vi "Drive Call.vi"(1 "Joystick Axes":dbl[](array[numeric]), 2 "Right Button Values":bool[](array[boolean]), 3 "Left Button Values":bool[](array[boolean])) -> ()   [LabVIEW 2018]
uses:
  Implementation/Drive Setpoints.ctl
  Implementation/Drive Operations.ctl
  <vilib>/Rock Robotics/Network Tables/NT Write Boolean.vi
  <vilib>/functionblocks/Edge Detection/One Shot Rising with Input/One Shot Rising with Input.vi
  <vilib>/functionblocks/FB Core/FB Core.xnode
  <vilib>/functionblocks/NI_FunctionBlock Libraries.lvlib
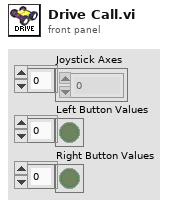
[diagram p1: front panel]
types:
  T1 = typedef "Drive Setpoints.ctl" = cluster{"Operation":T2, "Left Setpoint":dbl, "Right Setpoint":dbl, "Duration":dbl, "Enable Gyro Compensation":bool, "Gyro Turn Angle ":dbl}
  T2 = typedef "Drive Operations.ctl" = enum16{"Reserve", "Read Current", "Immediate", "Drive for Time", "Drive for Distance", "Gyro Turn"}
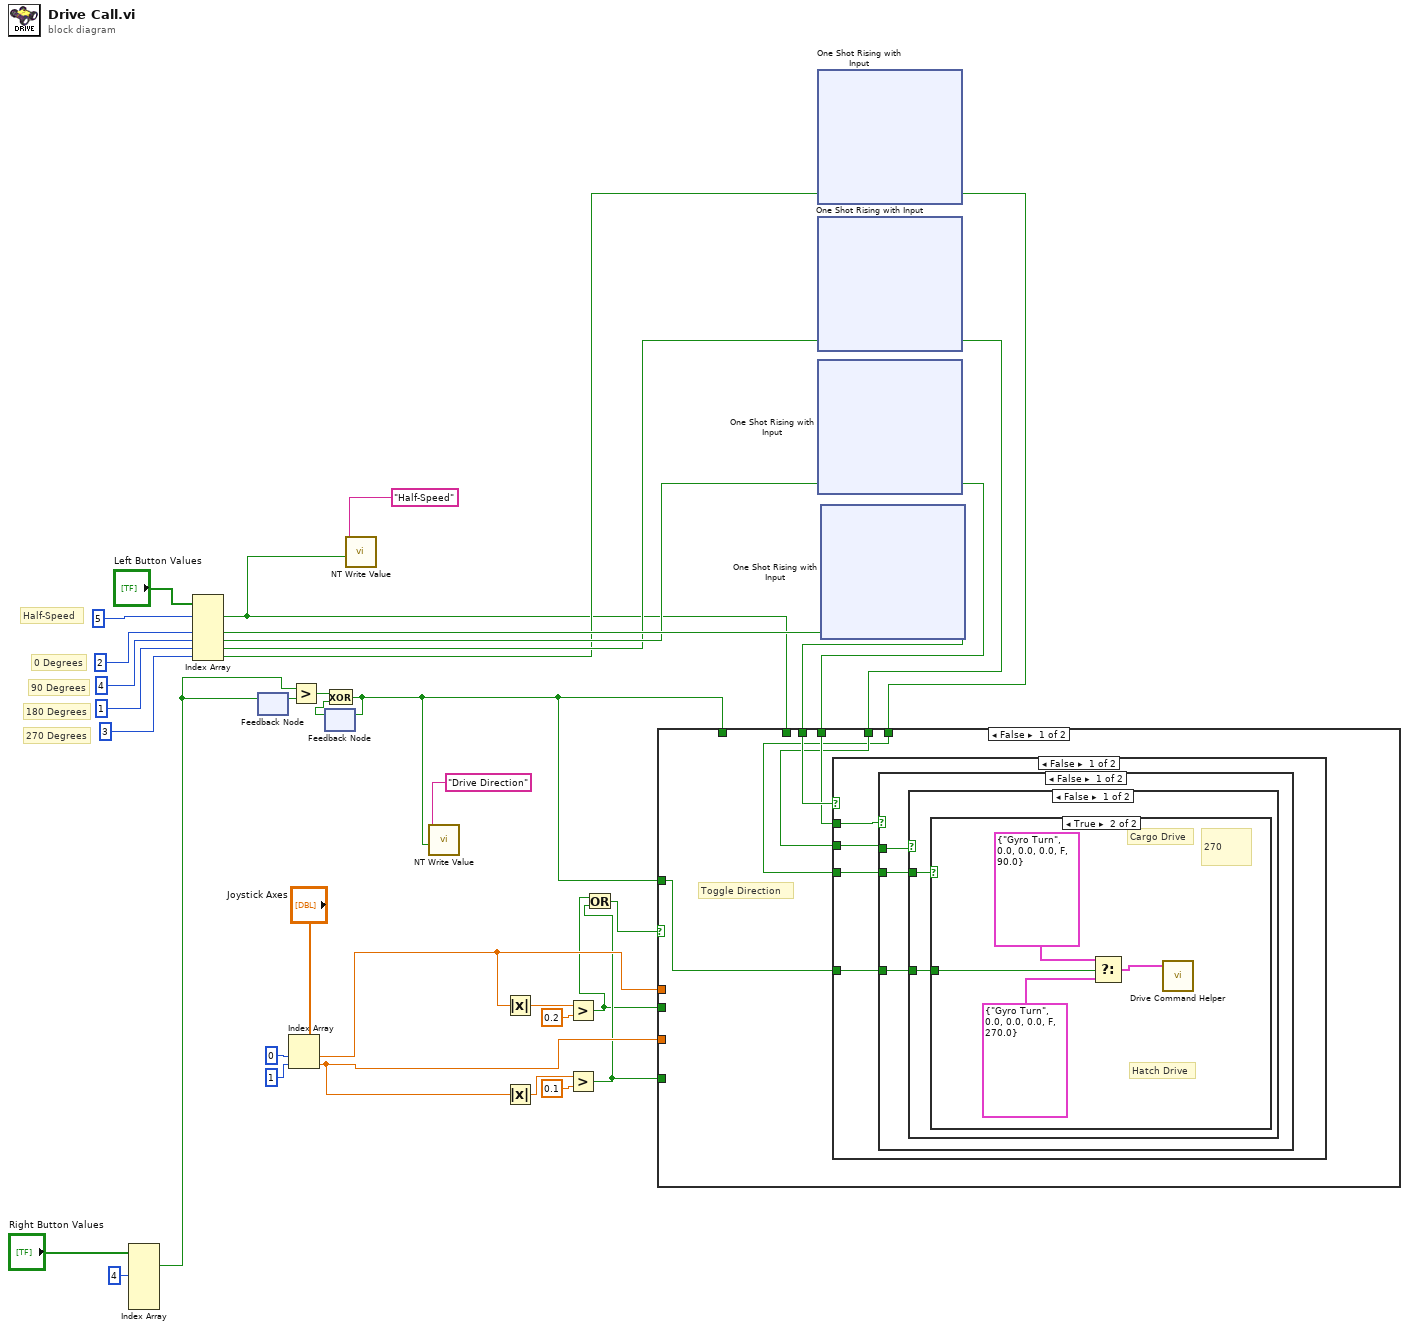
[diagram p0: block diagram]
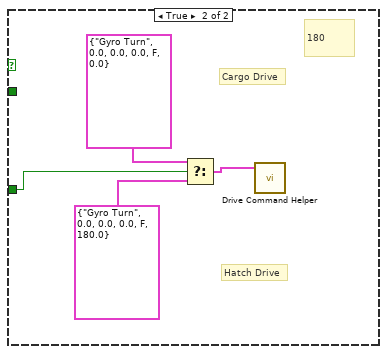
[diagram p3: hidden frame]
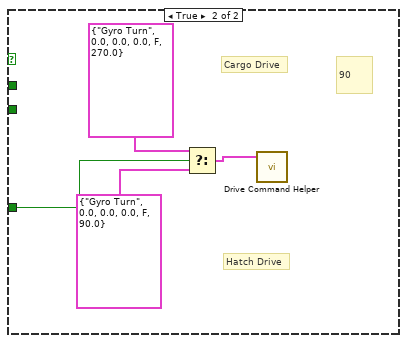
[diagram p4: hidden frame]
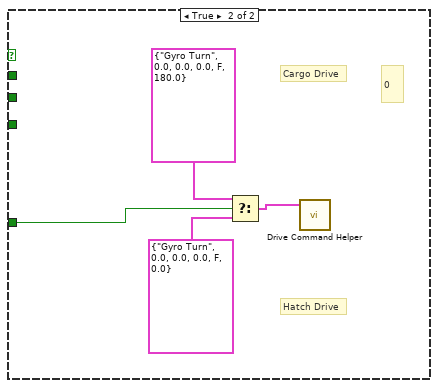
[diagram p5: hidden frame]
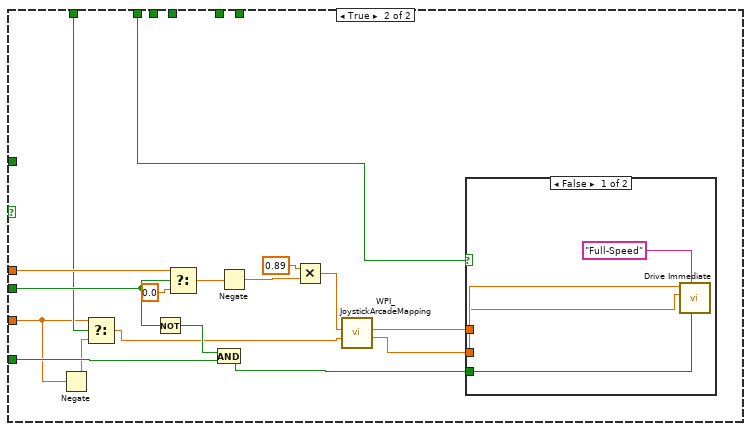
[diagram p6: hidden frame]
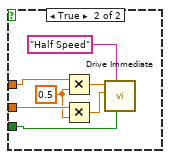
[diagram p7: hidden frame]
diagram:
  # "270 Degrees"
  # "180 Degrees"
  # "90 Degrees"
  # "0 Degrees"
  # "Half-Speed"
  n1 = Index Array(array="Right Button Values", index #1=4 ("index")) -> (element #1=w2:bool)  [unwired: 5 in, 5 out]
  n2 = Index Array(array="Left Button Values", index #1=5 ("index"), index #3=2 ("index"), index #4=4 ("index"), index #5=1 ("index"), index #6=3 ("index")) -> (element #1=w4:bool, element #3=w16:bool, element #4=w12:bool, element #5=w11:bool, element #6=w10:bool)  [unwired: 1 in, 1 out]
  n3 = feedback #1() -> (w25:bool)  [unwired: 1 in]
  n4 = feedback-in #1(w2) -> ()
  n5 = Index Array(array="Joystick Axes", index #1=0 ("index"), index #2=1 ("index")) -> (element #1=w27:dbl, element #2=w22:dbl)
  n6 = Greater?(x=w2, y=w25) -> (0:w26:bool)
  n7 = feedback #2() -> (w24:bool)  [unwired: 1 in]
  n8 = Exclusive Or(1:w24, 2:w26) -> (0:w9:bool)
  n9 = feedback-in #2(w9) -> ()
  n10 = call-poly <vilib>:"NT Write Value.vi"("Boolean"=w4, "Name"="Half-Speed") -> ()  [unwired: 9 in, 1 out]
  n11 = call-poly <vilib>:"NT Write Value.vi"("Boolean"=w9, "Name"="Drive Direction") -> ()  [unwired: 9 in, 1 out]
  n12 = Absolute Value(x=w27) -> (abs(x)=w31:dbl)
  n13 = Absolute Value(x=w22) -> (abs(x)=w29:dbl)
  n14 = Greater?(x=w31, y=0.2) -> (0:w20:bool)
  n15 = Greater?(x=w29, y=0.1) -> (0:w21:bool)
  n16 = Or(x=w20, y=w21) -> (x .or. y?=w19:bool)
  n17 = xnode "One Shot Rising with Input"("input"=w10) -> ("output"=w6:bool)  [unwired: 1 in, 1 out]
  n18 = xnode "One Shot Rising with Input"("input"=w11) -> ("output"=w7:bool)  [unwired: 1 in, 1 out]
  n19 = xnode "One Shot Rising with Input"("input"=w12) -> ("output"=w8:bool)  [unwired: 1 in, 1 out]
  n20 = xnode "One Shot Rising with Input"("input"=w16) -> ("output"=w17:bool)  [unwired: 1 in, 1 out]
  n21 = case shown="False" w19 {
    tunnel: w20 -> [_ w76]
    tunnel: w21 -> [_ w74]
    tunnel: w4 -> [_ w72]
    tunnel: w27 -> [_ w71]
    tunnel: w9 -> [_ w68]
    tunnel: w22 -> [_ w67]
    tunnel: w17 -> [w41 _]
    tunnel: w9 -> [w40 _]
    tunnel: w8 -> [w39 _]
    tunnel: w7 -> [w38 _]
    tunnel: w6 -> [w37 _]
    frame False {
      # "Toggle Direction"
      n22 = case shown="False" w41 {
        tunnel: w40 -> [w44 w63]
        tunnel: w39 -> [w45 _]
        tunnel: w38 -> [w43 _]
        tunnel: w37 -> [w42 _]
        frame False {
          n23 = case shown="False" w45 {
            tunnel: w44 -> [w48 w59]
            tunnel: w43 -> [w47 _]
            tunnel: w42 -> [w46 _]
            frame False {
              n24 = case shown="False" w47 {
                tunnel: w48 -> [w50 w55]
                tunnel: w46 -> [w49 _]
                frame False {
                  n25 = case shown="True" w49 {
                    tunnel: w50 -> [_ w51]
                    frame False {
                    }
                    frame True {
                      # "270"
                      # "Hatch Drive"
                      # "Cargo Drive"
                      n26 = Select(t=T1 {"Operation"=enum."Gyro Turn", "Left Setpoint"=0.0, "Right Setpoint"=0.0, "Duration"=0.0, "Enable Gyro Compensation"=FALSE, "Gyro Turn Angle "=90.0} ("SubSystem Data"), s=w51, f=T1 {"Operation"=enum."Gyro Turn", "Left Setpoint"=0.0, "Right Setpoint"=0.0, "Duration"=0.0, "Enable Gyro Compensation"=FALSE, "Gyro Turn Angle "=270.0} ("SubSystem Data")) -> (s? t:f=w53:T1)
                      n27 = call "Drive Command Helper.vi"("SubSystem Data"=w53) -> ()  [unwired: 8 in, 3 out]
                    }
                  }
                }
                frame True {
                  # "Hatch Drive"
                  # "Cargo Drive"
                  # "180"
                  n28 = Select(t=T1 {"Operation"=enum."Gyro Turn", "Left Setpoint"=0.0, "Right Setpoint"=0.0, "Duration"=0.0, "Enable Gyro Compensation"=FALSE, "Gyro Turn Angle "=0.0} ("SubSystem Data"), s=w55, f=T1 {"Operation"=enum."Gyro Turn", "Left Setpoint"=0.0, "Right Setpoint"=0.0, "Duration"=0.0, "Enable Gyro Compensation"=FALSE, "Gyro Turn Angle "=180.0} ("SubSystem Data")) -> (s? t:f=w57:T1)
                  n29 = call "Drive Command Helper.vi"("SubSystem Data"=w57) -> ()  [unwired: 8 in, 3 out]
                }
              }
            }
            frame True {
              # "Hatch Drive"
              # "Cargo Drive"
              # "90"
              n30 = Select(t=T1 {"Operation"=enum."Gyro Turn", "Left Setpoint"=0.0, "Right Setpoint"=0.0, "Duration"=0.0, "Enable Gyro Compensation"=FALSE, "Gyro Turn Angle "=270.0} ("SubSystem Data"), s=w59, f=T1 {"Operation"=enum."Gyro Turn", "Left Setpoint"=0.0, "Right Setpoint"=0.0, "Duration"=0.0, "Enable Gyro Compensation"=FALSE, "Gyro Turn Angle "=90.0} ("SubSystem Data")) -> (s? t:f=w61:T1)
              n31 = call "Drive Command Helper.vi"("SubSystem Data"=w61) -> ()  [unwired: 8 in, 3 out]
            }
          }
        }
        frame True {
          # "Hatch Drive"
          # "Cargo Drive"
          # "0"
          n32 = Select(t=T1 {"Operation"=enum."Gyro Turn", "Left Setpoint"=0.0, "Right Setpoint"=0.0, "Duration"=0.0, "Enable Gyro Compensation"=FALSE, "Gyro Turn Angle "=180.0} ("SubSystem Data"), s=w63, f=T1 {"Operation"=enum."Gyro Turn", "Left Setpoint"=0.0, "Right Setpoint"=0.0, "Duration"=0.0, "Enable Gyro Compensation"=FALSE, "Gyro Turn Angle "=0.0} ("SubSystem Data")) -> (s? t:f=w64:T1)
          n33 = call "Drive Command Helper.vi"("SubSystem Data"=w64) -> ()  [unwired: 8 in, 3 out]
        }
      }
    }
    frame True {
      n34 = Negate(x=w67) -> (-x=w70:dbl)
      n35 = Select(t=w67, s=w68, f=w70) -> (s? t:f=w69:dbl)
      n36 = Not(x=w76) -> (.not. x?=w75:bool)
      n37 = Select(t=w71, s=w76, f=0.0) -> (s? t:f=w81:dbl)
      n38 = And(x=w75, y=w74) -> (x .and. y?=w73:bool)
      n39 = Negate(x=w81) -> (-x=w79:dbl)
      n40 = Multiply(x=0.89, y=w79) -> (x*y=w77:dbl)
      n41 = call <vilib>:"WPI_JoystickArcadeMapping.vi"("Y axis value"=w69, "X axis value"=w77) -> ("Right Motor Value"=w82:dbl, "Left Motor Value"=w83:dbl)  [unwired: 8 in]
      n42 = case shown="False" w72 {
        tunnel: w83 -> [w87 w94]
        tunnel: w82 -> [w86 w93]
        tunnel: w73 -> [w84 w88]
        frame False {
          n43 = call "Drive Immediate.vi"("Enable Gyro Compensation"=w84, "Description"="Full-Speed", "Right Setpoint"=w86, "Left Setpoint"=w87) -> ()  [unwired: 7 in, 1 out]
        }
        frame True {
          w92 = 0.5 ("y")
          n44 = Multiply(x=w94, y=w92) -> (x*y=w90:dbl)
          n45 = Multiply(x=w93, y=w92) -> (x*y=w91:dbl)
          n46 = call "Drive Immediate.vi"("Enable Gyro Compensation"=w88, "Description"="Half Speed", "Right Setpoint"=w91, "Left Setpoint"=w90) -> ()  [unwired: 7 in, 1 out]
        }
      }
    }
  }
